vi "CalPoPup.vi"(5 "error in (no error)":errorcluster, 9 "Enable(t)":bool, 11 "RunCALvi(t)":bool) -> (10 "Success?(t)":bool, 19 "error out":errorcluster)   [LabVIEW 2018]
uses:
  <vilib>/Utility/miscctls.llb/LVRectTypeDef.ctl
  Initialize References/Sequence Globals.vi
panel:
  out "OK [CLOSE}":bool
  in  "ABORT":bool
  in  "ReStart":bool
  in  "Tab Control":enum32{"Pic1", "Pic2", "CalTab", "Help"}(tab)
  out "Front Panel Window:Panel Bounds":T1={"Left"=387, "Top"=289, "Right"=1039, "Bottom"=927}
  out "vi reference":refnum<vi>
  in  "Support_Path":path=path "C:/RageATE-Tetra/Automated Tests/Tetra WAM/Utilities/Cal Utilities/PNA_CalFile_Check.vi"
  in  "next":bool
  # "PRESS ABORT TO END"
  # "PRESS NEXT TO CONTINUE"
  # "Keysight PNA and E-Cal (N-4692A)"
  # ">>> Connect the E-Cal USB Cable to the PNA Front Panel USB port"
  # ">>> Connect the  RF Cable to PORT A"
  # "Instructions:"
  # "1. Connect the Ref Cable (1) \n    to \"PORT A\" on the E-Cal (2)       \n    Using an 8 in/lbTorque Wrench"
  # "2. Make Sure the \"READY\"\n    Indicator (3) is lit GREEN.\n    If the lamp is RED, wait up to \n    15 minutes"
  # "PRESS NEXT TO CONTINUE"
  # "### CAL SETTINGS. USER SHOULD NOT CHANGE !!"
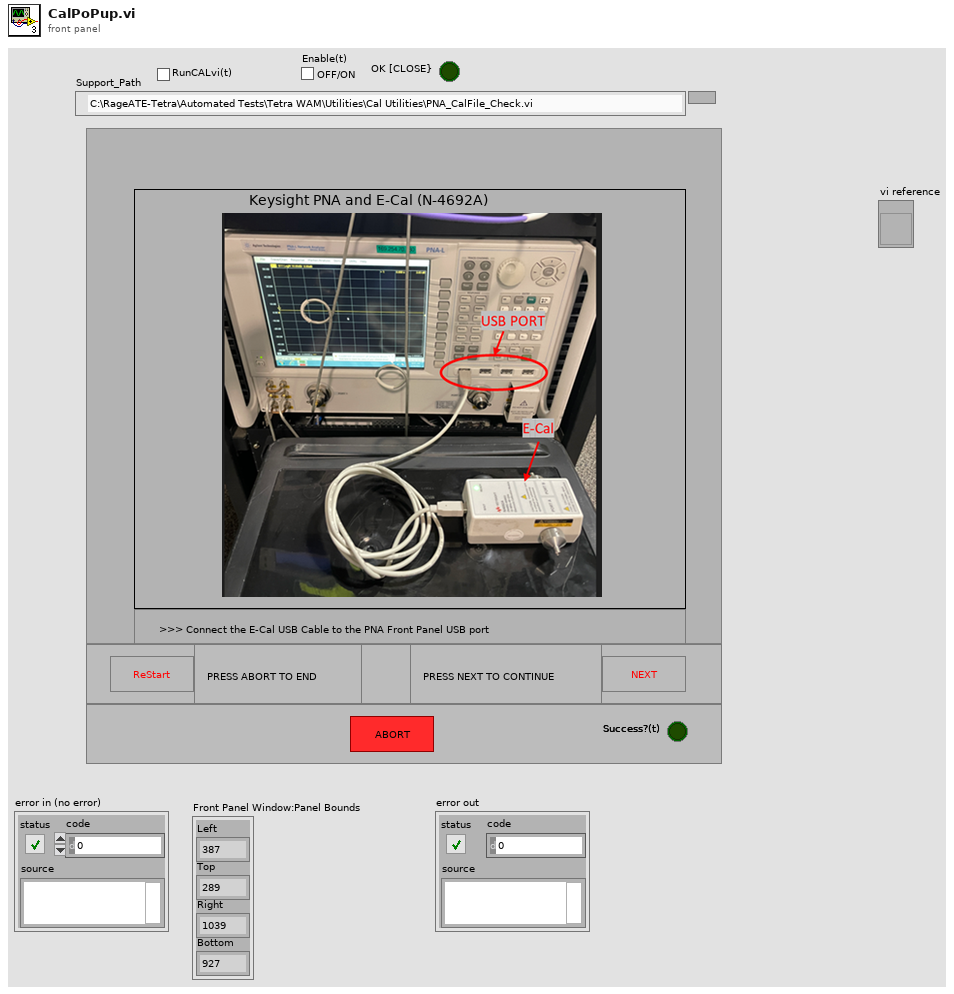
[diagram p1: front panel]
types:
  T1 = typedef "LVRectTypeDef.ctl" = cluster{"Left":i16, "Top":i16, "Right":i16, "Bottom":i16}
  T2 = enum32{"Invalid", "Standard", "Closed", "Hidden", "Minimized", "Maximized"}
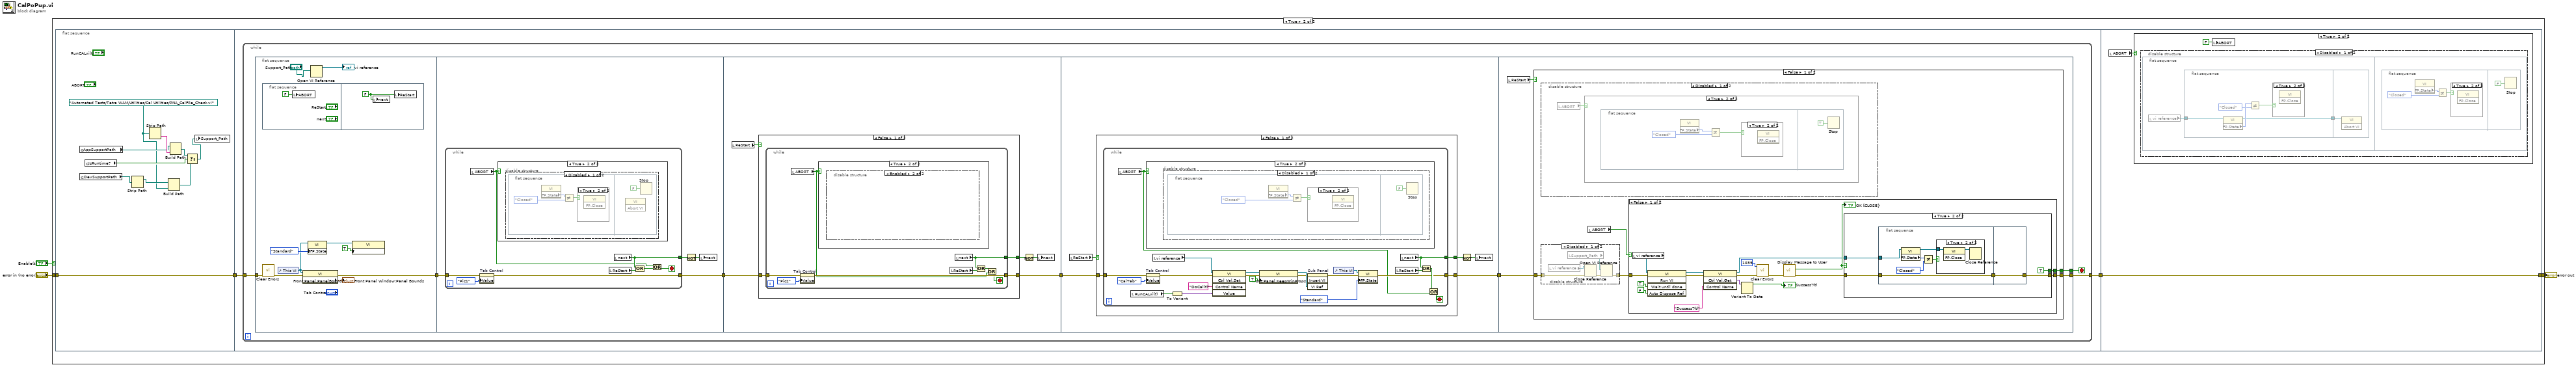
[diagram p0: block diagram]
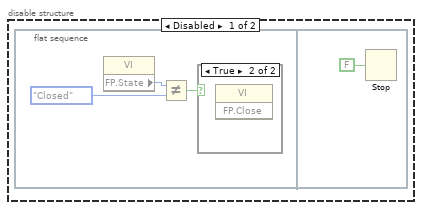
[diagram p7: hidden frame]
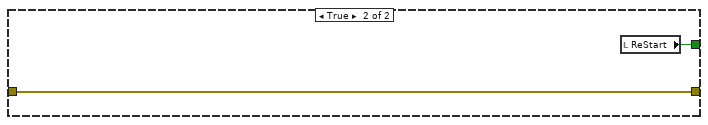
[diagram p9: hidden frame]
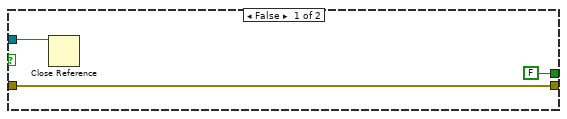
[diagram p14: hidden frame]
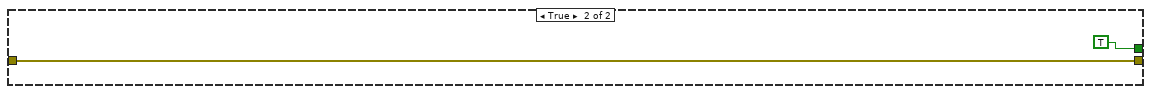
[diagram p16: hidden frame]
diagram:
  n1 = case shown="True" "Enable(t)" {
    tunnel: "error in (no error)" -> [w4 w8]
    tunnel: [w4 w7] -> w1
    frame False {
    }
    frame True {
      n2 = flat-sequence {
        tunnel: w8 -> [w18]
        tunnel: [w18] -> w5
        tunnel: [w19] -> w6
        tunnel: w5 -> [w20]
        tunnel: [w172] -> w7
        tunnel: w6 -> [w172]
        frame #0 {
          w10 = path "Automated Tests/Tetra WAM/Utilities/Cal Utilities/PNA_CalFile_Check.vi" ("vi path")
          n3 = global read "Sequence Globals.vi" "AppSupportPath"() -> (w16:path)
          n4 = global read "Sequence Globals.vi" "DevSupportPath"() -> (w12:path)
          n5 = global read "Sequence Globals.vi" "IsRuntime?"() -> (w14:bool)
          n6 = Strip Path(path=w12) -> (stripped path=w11:path)  [unwired: 1 out]
          n7 = Strip Path(path=w10) -> (name=w17:string)  [unwired: 1 out]
          n8 = Build Path(base path=w11, name or relative path=w10) -> (appended path=w9:path)
          n9 = Build Path(base path=w16, name or relative path=w17) -> (appended path=w15:path)
          n10 = Select(t=w15, s=w14, f=w9) -> (s? t:f=w13:path)
          n11 = local write "Support_Path"(w13) -> ()
        }
        frame #1 {
          n12 = while {
            tunnel: w20 -> [w23]
            tunnel: [w22] -> w19
            stop <- w21 stop-if-true
            n13 = flat-sequence {
              tunnel: [w34] -> w27
              tunnel: w23 -> [w31]
              tunnel: w27 -> [w41]
              tunnel: [w40] -> w26
              tunnel: w26 -> [w59]
              tunnel: [w57] -> w25
              tunnel: w25 -> [w82]
              tunnel: [w80] -> w24
              tunnel: w24 -> [w116]
              tunnel: [w114] -> w21
              tunnel: [w113] -> w22
              frame #0 {
                n14 = flat-sequence {
                  frame #0 {
                    n15 = local write "ABORT"(FALSE ("ABORT")) -> ()
                  }
                  frame #1 {
                    w39 = FALSE
                    n16 = local write "next"(w39) -> ()
                    n17 = local write "ReStart"(w39) -> ()
                  }
                }
                n18 = call <vilib>:"Clear Errors.vi"("error in (no error)"=w31) -> ("error out"=w30:errorcluster)  [unwired: 5 in, 1 out]
                n19 = control-ref of="This VI"() -> (w33:refnum<vi>)
                n20 = property class="VI"(reference=w33, error in=w30) -> (error out=w34:errorcluster, "Front Panel.PanelBounds"=→"Front Panel Window:Panel Bounds":T1)  [unwired: 1 out]
                n21 = property class="VI"(reference=w33, "FP.State"=T2."Standard" ("Front Panel Window:State")) -> (reference out=w36:refnum<vi>)  [unwired: 1 in, 1 out]
                n22 = Open VI Reference(vi path="Support_Path") -> (vi reference=→"vi reference":refnum<vi>)  [unwired: 5 in, 1 out]
                n23 = property class="VI"(reference=w36, "Front Panel.IsFrontmost"=TRUE ("Front Panel Window:Is Frontmost")) -> ()  [unwired: 1 in, 2 out]
              }
              frame #1 {
                n24 = while {
                  tunnel: [w46] -> w43
                  tunnel: [w50] -> w40
                  tunnel: w41 -> [w49]
                  stop <- w45 stop-if-true
                  n25 = local read "ABORT"() -> (w44:bool)
                  n26 = property on="Tab Control" class="TabCtl (strict)"(error in=w49, "Value"=enum32{"Pic1", "Pic2", "CalTab", "Help"}."Pic1" ("Tab Control")) -> (error out=w50:errorcluster)  [unwired: 1 in, 1 out]
                  n27 = case shown="True" w44 {
                    frame False {
                    }
                    frame True {
                      n28 = disable-structure shown="Disabled" {
                        frame Disabled {
                          n29 = flat-sequence {
                            frame #0 {
                              n30 = property class="VI"() -> ("FP.State"=w54:T2)  [unwired: 2 in, 2 out]
                              n31 = Not Equal?(x=w54, y=T2."Closed") -> (x != y?=w52:bool)
                              n32 = case shown="True" w52 {
                                frame False {
                                }
                                frame True {
                                n33 = invoke class="VI" method="FP.Close"() -> ()  [unwired: 3 in, 3 out]
                                }
                              }
                            }
                            frame #1 {
                              n34 = invoke class="VI" method="Abort VI"() -> ()  [unwired: 3 in, 3 out]
                              n35 = Stop(stop? (T)=FALSE) -> ()
                            }
                          }
                        }
                        frame Enabled {
                        }
                      }
                    }
                  }
                  n36 = local read "ReStart"() -> (w48:bool)
                  n37 = local read "next"() -> (w46:bool)
                  n38 = Or(x=w46, y=w48) -> (x .or. y?=w47:bool)
                  n39 = Or(x=w44, y=w47) -> (x .or. y?=w45:bool)
                }
                n40 = Not(x=w43) -> (.not. x?=w42:bool)
                n41 = local write "next"(w42) -> ()
              }
              frame #2 {
                n42 = local read "ReStart"() -> (w56:bool)
                n43 = case shown="False" w56 {
                  tunnel: w59 -> [w63 w77]
                  tunnel: [w62 w77] -> w57
                  tunnel: [w61 w76] -> w58
                  frame False {
                    n44 = while {
                      tunnel: [w66] -> w61
                      tunnel: [w70] -> w62
                      tunnel: w63 -> [w69]
                      stop <- w65 stop-if-true
                      n45 = local read "ABORT"() -> (w64:bool)
                      n46 = property on="Tab Control" class="TabCtl (strict)"(error in=w69, "Value"=enum32{"Pic1", "Pic2", "CalTab", "Help"}."Pic2" ("Tab Control")) -> (error out=w70:errorcluster)  [unwired: 1 in, 1 out]
                      n47 = case shown="True" w64 {
                        frame False {
                        }
                        frame True {
                          n48 = disable-structure shown="Enabled" {
                            frame Disabled {
                              n49 = flat-sequence {
                                frame #0 {
                                n50 = property class="VI"() -> ("FP.State"=w74:T2)  [unwired: 2 in, 2 out]
                                n51 = Not Equal?(x=w74, y=T2."Closed") -> (x != y?=w72:bool)
                                n52 = case shown="True" w72 {
                                frame False {
                                }
                                frame True {
                                n53 = invoke class="VI" method="FP.Close"() -> ()  [unwired: 3 in, 3 out]
                                }
                                }
                                }
                                frame #1 {
                                n54 = Stop(stop? (T)=FALSE) -> ()
                                }
                              }
                            }
                            frame Enabled {
                            }
                          }
                        }
                      }
                      n55 = local read "ReStart"() -> (w67:bool)
                      n56 = local read "next"() -> (w66:bool)
                      n57 = Or(x=w66, y=w67) -> (x .or. y?=w68:bool)
                      n58 = Or(x=w68, y=w64) -> (x .or. y?=w65:bool)
                    }
                  }
                  frame True {
                    n59 = local read "ReStart"() -> (w76:bool)
                  }
                }
                n60 = Not(x=w58) -> (.not. x?=w60:bool)
                n61 = local write "next"(w60) -> ()
              }
              frame #3 {
                n62 = local read "ReStart"() -> (w78:bool)
                n63 = case shown="False" w78 {
                  selector: w78 -> [_ w111]
                  tunnel: w82 -> [w85 w112]
                  tunnel: [w84 w111] -> w79
                  tunnel: [w83 w112] -> w80
                  frame False {
                    n64 = while {
                      tunnel: [w88] -> w84
                      tunnel: w85 -> [w105]
                      tunnel: [w98] -> w83
                      stop <- w87 stop-if-true
                      n65 = local read "ABORT"() -> (w86:bool)
                      n66 = local read "RunCALvi(t)"() -> (w96:bool)
                      n67 = case shown="True" w86 {
                        frame False {
                        }
                        frame True {
                          n68 = disable-structure shown="Disabled" {
                            frame Disabled {
                              n69 = flat-sequence {
                                frame #0 {
                                n70 = property class="VI"() -> ("FP.State"=w109:T2)  [unwired: 2 in, 2 out]
                                n71 = Not Equal?(x=w109, y=T2."Closed") -> (x != y?=w107:bool)
                                n72 = case shown="True" w107 {
                                frame False {
                                }
                                frame True {
                                n73 = invoke class="VI" method="FP.Close"() -> ()  [unwired: 3 in, 3 out]
                                }
                                }
                                }
                                frame #1 {
                                n74 = Stop(stop? (T)=FALSE) -> ()
                                }
                              }
                            }
                            frame Enabled {
                            }
                          }
                        }
                      }
                      n75 = property on="Tab Control" class="TabCtl (strict)"(error in=w105, "Value"=enum32{"Pic1", "Pic2", "CalTab", "Help"}."CalTab" ("Tab Control")) -> (error out=w92:errorcluster)  [unwired: 1 in, 1 out]
                      n76 = local read "vi reference"() -> (w93:refnum<vi>)
                      n77 = To Variant(anything=w96) -> (Variant=w91:variant)
                      n78 = invoke class="VI" method="Ctrl Val.Set"(reference=w93, error in=w92, "Control Name"="DoCal(t)", "Value"=w91) -> (reference out=w94:refnum<vi>, error out=w90:errorcluster)  [unwired: 1 in, 3 out]
                      n79 = property class="VI"(reference=w94, error in=w90, "Front Panel.KeepWinProps"=TRUE ("Front Panel Window:Keep Window Proportions")) -> (reference out=w102:refnum<vi>, error out=w101:errorcluster)
                      n80 = invoke on="Sub Panel" class="SubPnl" method="Insert VI"(error in=w101, "VI Ref"=w102) -> (error out=w99:errorcluster)  [unwired: 2 in, 3 out]
                      n81 = control-ref of="This VI"() -> (w89:refnum<vi>)
                      n82 = property class="VI"(reference=w89, error in=w99, "FP.State"=T2."Standard" ("Front Panel Window:State")) -> (error out=w98:errorcluster)  [unwired: 1 out]
                      n83 = local read "ReStart"() -> (w103:bool)
                      n84 = local read "next"() -> (w88:bool)
                      n85 = Or(x=w88, y=w103) -> (x .or. y?=w104:bool)
                      n86 = Or(x=w104, y=w86) -> (x .or. y?=w87:bool)
                    }
                  }
                  frame True {
                  }
                }
                n87 = Not(x=w79) -> (.not. x?=w81:bool)
                n88 = local write "next"(w81) -> ()
              }
              frame #4 {
                n89 = local read "ReStart"() -> (w115:bool)
                n90 = case shown="False" w115 {
                  tunnel: w116 -> [w119 w170]
                  tunnel: [w121 w170] -> w113
                  tunnel: [w120 w168] -> w114
                  frame False {
                    n91 = disable-structure shown="Disabled" {
                      frame Disabled {
                        n92 = local read "ABORT"() -> (w163:bool)
                        n93 = case shown="True" w163 {
                          frame False {
                          }
                          frame True {
                            n94 = flat-sequence {
                              frame #0 {
                                n95 = property class="VI"() -> ("FP.State"=w166:T2)  [unwired: 2 in, 2 out]
                                n96 = Not Equal?(x=w166, y=T2."Closed") -> (x != y?=w164:bool)
                                n97 = case shown="True" w164 {
                                frame False {
                                }
                                frame True {
                                n98 = invoke class="VI" method="FP.Close"() -> ()  [unwired: 3 in, 3 out]
                                }
                                }
                              }
                              frame #1 {
                                n99 = Stop(stop? (T)=TRUE) -> ()
                              }
                            }
                          }
                        }
                      }
                      frame Enabled {
                      }
                    }
                    n100 = disable-structure shown="Disabled" {
                      disable-tunnel: w119 -> [w160 _]
                      disable-tunnel: [w158 _] -> w118
                      frame Disabled {
                        n101 = local read "vi reference"() -> (w162:refnum<vi>)
                        n102 = local read "Support_Path"() -> (w159:path)
                        n103 = Close Reference(reference=w162, error in (no error)=w160) -> (error out=w161:errorcluster)
                        n104 = Open VI Reference(vi path=w159, error in (no error)=w161) -> (error out=w158:errorcluster)  [unwired: 4 in, 1 out]
                      }
                      frame Enabled {
                      }
                    }
                    n105 = local read "ABORT"() -> (w117:bool)
                    n106 = case shown="False" w117 {
                      tunnel: [w137 w157] -> w121
                      tunnel: [w134 TRUE] -> w120
                      tunnel: w118 -> [w129 w157]
                      frame False {
                        n107 = local read "vi reference"() -> (w130:refnum<vi>)
                        n108 = invoke class="VI" method="Run VI"(reference=w130, error in=w129, "Wait until done"=TRUE ("Wait Until Done"), "Auto Dispose Ref"=FALSE ("Auto Dispose Reference")) -> (reference out=w127:refnum<vi>, error out=w126:errorcluster)  [unwired: 1 in, 3 out]
                        n109 = invoke class="VI" method="Ctrl Val.Get"(reference=w127, error in=w126, "Control Name"="Success?(t)") -> (reference out=w123:refnum<vi>, error out=w125:errorcluster, "Get Control Value Variant"=w124:variant)  [unwired: 1 in, 1 out]
                        n110 = Variant To Data(Variant=w124) -> (data=→"Success?(t)":bool)  [unwired: 2 in, 1 out]
                        n111 = call <vilib>:"Clear Errors.vi"("error in (no error)"=w125, "specific error code to clear (0: all)"=1039) -> ("error out"=w133:errorcluster)  [unwired: 4 in, 1 out]
                        n112 = call "Display Message to User"("error in (no error)"=w133) -> ("error out"=w135:errorcluster, "OK [CLOSE}"=w136:bool)  [unwired: 9 in]
                        "OK [CLOSE}" <- w136
                        n113 = case shown="True" w136 {
                          tunnel: w135 -> [w141 w143]
                          tunnel: [w141 w145] -> w137
                          tunnel: [FALSE TRUE] -> w134
                          tunnel: w123 -> [w139 w142]
                          frame False {
                            n114 = Close Reference(reference=w139) -> ()  [unwired: 1 in, 1 out]
                          }
                          frame True {
                            n115 = flat-sequence {
                              tunnel: [w149] -> w144
                              tunnel: w143 -> [w149]
                              tunnel: w142 -> [w147]
                              tunnel: [w155] -> w145
                              tunnel: w144 -> [w155]
                              frame #0 {
                                n116 = property class="VI"(reference=w147) -> (reference out=w148:refnum<vi>, "FP.State"=w152:T2)  [unwired: 1 in, 1 out]
                                n117 = Not Equal?(x=w152, y=T2."Closed") -> (x != y?=w150:bool)
                                n118 = case shown="True" w150 {
                                tunnel: w148 -> [_ w153]
                                frame False {
                                }
                                frame True {
                                n119 = invoke class="VI" method="FP.Close"(reference=w153) -> (reference out=w154:refnum<vi>)  [unwired: 2 in, 2 out]
                                n120 = Close Reference(reference=w154) -> ()  [unwired: 1 in, 1 out]
                                }
                                }
                              }
                              frame #1 {
                              }
                            }
                          }
                        }
                      }
                      frame True {
                      }
                    }
                  }
                  frame True {
                    n121 = call "Display Message to User2"() -> ("YES"=w169:bool)  [unwired: 10 in, 1 out]
                    n122 = Not(x=w169) -> (.not. x?=w168:bool)
                  }
                }
              }
            }
          }
        }
        frame #2 {
          n123 = local read "ABORT"() -> (w171:bool)
          n124 = case shown="True" w171 {
            frame False {
              n125 = flat-sequence {
                frame #0 {
                  n126 = property class="VI"() -> ("FP.State"=w175:T2)  [unwired: 2 in, 2 out]
                  n127 = Not Equal?(x=w175, y=T2."Closed") -> (x != y?=w173:bool)
                  n128 = case shown="True" w173 {
                    frame False {
                    }
                    frame True {
                      n129 = invoke class="VI" method="FP.Close"() -> ()  [unwired: 3 in, 3 out]
                    }
                  }
                }
                frame #1 {
                  n130 = Stop(stop? (T)=FALSE) -> ()
                }
              }
            }
            frame True {
              n131 = disable-structure shown="Disabled" {
                frame Disabled {
                  n132 = flat-sequence {
                    frame #0 {
                      n133 = local read "vi reference"() -> (w178:refnum<vi>)
                      n134 = flat-sequence {
                        tunnel: [w181] -> w179
                        tunnel: w178 -> [w180]
                        tunnel: w179 -> [w185]
                        frame #0 {
                          n135 = property class="VI"(reference=w180) -> (reference out=w181:refnum<vi>, "FP.State"=w184:T2)  [unwired: 1 in, 1 out]
                          n136 = Not Equal?(x=w184, y=T2."Closed") -> (x != y?=w182:bool)
                          n137 = case shown="True" w182 {
                            frame False {
                            }
                            frame True {
                              n138 = invoke class="VI" method="FP.Close"() -> ()  [unwired: 3 in, 3 out]
                            }
                          }
                        }
                        frame #1 {
                          n139 = invoke class="VI" method="Abort VI"(reference=w185) -> ()  [unwired: 2 in, 3 out]
                        }
                      }
                    }
                    frame #1 {
                      n140 = flat-sequence {
                        frame #0 {
                          n141 = property class="VI"() -> ("FP.State"=w188:T2)  [unwired: 2 in, 2 out]
                          n142 = Not Equal?(x=w188, y=T2."Closed") -> (x != y?=w186:bool)
                          n143 = case shown="True" w186 {
                            frame False {
                            }
                            frame True {
                              n144 = invoke class="VI" method="FP.Close"() -> ()  [unwired: 3 in, 3 out]
                            }
                          }
                        }
                        frame #1 {
                          n145 = Stop(stop? (T)=FALSE) -> ()
                        }
                      }
                    }
                  }
                }
                frame Enabled {
                }
              }
              n146 = local write "ABORT"(FALSE ("ABORT")) -> ()
            }
          }
        }
      }
    }
  }
  "error out" <- w1
